vi "SubVI_Strain_test.vi"() -> (0 "error out":errorcluster caption="에러 출력", 3 "웨이브폼 차트":waveform(dbl)[](graph)=[{"t0"=timestamp(3537999110.3911605 s since 1904-01-01), "dt"=0.00062, "Y"=[0.00047262587047964, 0.00041043910651785673, 0.0005114070256648253, 0.0004353033393431034, 0.0004534332939897456, 0.000463390432462872, 0.00043454570170866036, 0.0003840550210499824, 0.00046049693560497513, 0.00043601921847729236, 0.00038526592644869665, 0.0005006792607078738, 0.00047117014412360745, 0.0004275898066649711, 0.00042875309283979117, 0.0004913538098973309, 0.00038979939141159815, 0.00047844285209712467, 0.00036011787223929454, 0.0004068360428684548, 0.0004042828942719733, 0.0004761339497591499, 0.0003612452128748545, 0.00039843694890317436, 0.0004418536716216596, 0.00036188344388491333, 0.0004565713521915321, 0.00047409353330743514, 0.00037547139637794424, 0.00033699303793574255, 0.00041919632967674477, 0.0004044857140110813, 0.0003804044274407727, 0.0004687777505846543, 0.00042779860142021844, 0.00037995705260560905, 0.0003900678215465565, 0.0004465785547122237, 0.00037223244355367514, 0.0004662123537668788, 0.00045247278961574056, 0.0003887435676117308, 0.0003601775198283073, 0.00036035646263802423, 0.0003362236202489259, 0.00044848164523168013, 0.0003231198433927978, 0.00034800359433781783, 0.0003373986229292269, 0.00041982270369339325, 0.0003728468289415956, 0.00030865658295483727, 0.0004351243697196373, 0.00039441044463494316, 0.00040742660946971977, 0.0003725068291676455, 0.00034785447900801964, 0.00036742475482860114, 0.0003175730590198825, 0.00037625876929430786, 0.00034030930135528964, 0.0002938836142782422, 0.0003432021030489953, 0.0003697689446748764, 0.0003789907243272393, 0.0002950167696174689, 0.00037915774389622395, 0.00037210121570454955, 0.0003386332733897068, 0.0004143583625068418, 0.00033167274759207834, 0.0002777215202054256, 0.00035874597965521654, 0.00037385489980525907, 0.0003248852844424059, 0.00036311815478616875, 0.0002994301359364881, 0.000380660922526737, 0.0003066943831403147, 0.00029233298481648196, 0.00039809096652279293, 0.0002827788278151317, 0.0002551908820106478, 0.0003740815669064443, 0.00027501397323419517, 0.00037588297752052364, 0.00038506311450266543, 0.00026713592984576207, 0.0003405777049319909, 0.00025879285341093864, 0.0003032650250487586, 0.0003875087934527209, 0.00035051470316939084, 0.0002406520624579295, 0.00026611018313775064, 0.0003136366687181668, 0.00036281395036811534, 0.0003465422660227054, 0.0003349531889845697, 0.00034369716151030395], "attributes"=variant("NI_ChannelName"=variant(string "Strain/ai0"), "NI_UnitDescription"=variant(string "Strain"))}, {"t0"=timestamp(3537999110.3911605 s since 1904-01-01), "dt"=0.00062, "Y"=[0.0002669331657947935, 0.00031134641952601326, 0.0002354460989940313, 0.00016687317361001626, 0.00022731822544217194, 0.00024163601353161676, 0.0002590850674601926, 0.00023137916409462781, 0.00026835251587787164, 0.00026616981951666294, 0.00017885188772679905, 0.00017816022694101572, 0.00017185781023223087, 0.00017636549091540666, 0.0002635517891786011, 0.00022700814043906276, 0.00023874379922674913, 0.00024052683246014774, 0.00024122454284711817, 0.00016479228139494308, 0.00021975697672062318, 0.00028465743977653437, 0.0001807718476799469, 0.00022712740387904418, 0.00019713950741664365, 0.0002739703191745871, 0.00017310397715106191, 0.00017920964368102032, 0.00026575236501360995, 0.00014409711692620224, 0.00016225825528964416, 0.00019742572262577832, 0.0002141517083944936, 0.00023250025135162307, 0.00022681731899424989, 0.0002503843181970984, 0.0002561748616886476, 0.00020925609458375476, 0.00011095444145538343, 0.0002301745944171381, 0.00011181890140260174, 0.00010877839372105932, 0.00010601810569876974, 0.00023378831215355343, 0.00018893474107480976, 0.00016091671725580725, 0.0001314395631869098, 0.00024415851512703387, 0.00021396089185510105, 0.0001720724607719918, 0.00016615171716228845, 0.00011148504083206682, 0.00011351801668865663, 0.00010659639372036722, 0.0002298346916171518, 0.00013468291901361026, 0.0001456949844501603, 0.00021809924188589055, 0.00021406226313258812, 0.00014225480585682522, 0.00013101029708028974, 0.00013037236063033694, 0.0001637250076583648, 7.379600007796863e-05, 0.0001839439715783761, 0.0001691389113699347, 0.0001081583708945824, 0.00011124060734140677, 9.396363549484408e-05, 0.00014283313578525048, 0.00019245871942893576, 5.996587190824817e-05, 0.00020705576732404593, 7.412983548600947e-05, 5.854711315164868e-05, 8.0228332253737e-05, 5.655608874399001e-05, 0.00018115941812987514, 0.00017679479595671208, 6.82519803505827e-05, 0.00014493778539749518, 0.00010855184682994629, 0.00017683057139345637, 8.758478021039626e-05, 0.00012452961605176617, 0.00010902878777275229, 0.00017910827946800666, 5.026116552805535e-05, 0.00012914418620521909, 0.0001243746053905065, 0.0001760554375036641, 0.00014819315323548205, 0.00015514516356190044, 6.678550799302241e-05, 0.00016331360107205736, 8.419269311144614e-05, 4.2714515443818715e-05, 0.00010017564567018714, 0.0001209763068135592, 0.00010350226250175502], "attributes"=variant("NI_ChannelName"=variant(string "Strain/ai1"), "NI_UnitDescription"=variant(string "Strain"))}, {"t0"=timestamp(3537999110.3911605 s since 1904-01-01), "dt"=0.00062, "Y"=[7.764108211699364e-05, 1.4484139330982968e-05, 0.00010107585700148278, 6.181040236646698e-06, 8.555787126842158e-05, -1.462080646377688e-05, 6.060371854331264e-05, 7.160223008400242e-05, 4.869340815177723e-05, 3.8333218719135346e-05, 2.0105052086062475e-05, 8.583143028958988e-06, -2.0879072364570083e-05, 8.161734533826009e-05, 3.134110632507873e-05, -5.908855668863389e-05, -1.764266463601186e-05, -5.6490094374337585e-05, -3.236427656186244e-05, -5.9529578768390715e-05, 1.3631768895227626e-05, 2.8605088960366313e-05, 3.01727833530734e-05, -6.644880668367357e-05, -6.587667777447305e-05, 2.3973564275569672e-05, 5.4213366584198175e-05, 5.71104749832485e-05, 1.7214118757940295e-05, 5.4776971863549126e-06, 1.532458992461321e-05, -3.504034488329816e-05, -4.5231921596921784e-05, 4.3996126504963626e-05, -6.430331989833602e-05, -6.589455681279568e-05, -3.6667435101351785e-05, -3.8342200088792025e-05, -5.96785726263405e-05, 2.0897826413855974e-05, -5.958917631689875e-05, -1.1855224004457564e-05, 1.3280092006003315e-05, -3.2638440121926624e-05, -2.9270985978232148e-05, -8.310581447828447e-05, -9.599599094708993e-05, 7.420833785214426e-06, -6.753942560329031e-05, -8.866001355790166e-05, -6.653224209489772e-05, 2.3121177662968224e-05, 3.486884085512345e-06, -3.879516047389555e-05, 5.126002383805686e-07, -9.907099088208958e-05, -3.235235640366676e-05, -6.12400255867085e-05, -6.194923352693948e-05, -0.00011208589745393728, -0.0001289916598464899, -4.500544437136647e-05, -0.00013066611559436767, -0.00010190760195845445, -7.196743317198027e-05, -3.4056936140276524e-05, -3.583303052276851e-05, -0.00013141693734695874, -2.2035352919422305e-05, -2.1081719665376785e-05, -0.00010476803380497741, -3.408673643363535e-05, -9.041943393893871e-06, -4.126855533843273e-05, -5.5751079689928154e-05, -0.00010771783700580792, -2.5605501263270295e-05, -0.00011601890695171023, -0.00014168401373086987, -0.0001582491364176448, -0.00012089341214936181, -4.6745740417333314e-05, -4.3968415765053384e-05, -4.3509500120545156e-05, -4.439157137568061e-05, -0.00010854020328056746, -0.0001660369378640863, -6.683618526089393e-05, -8.957776154292598e-05, -9.402941130561796e-05, -7.741448424702261e-05, -0.0001709764980914279, -0.0001377452473136861, -0.0001570097505522338, -0.00010712191857012992, -0.00018182071726395756, -5.1769917274699954e-05, -0.00015633642905843735, -8.77243856311545e-05, -5.209770879092542e-05], "attributes"=variant("NI_ChannelName"=variant(string "Strain/ai2"), "NI_UnitDescription"=variant(string "Strain"))}, {"t0"=timestamp(3537999110.3911605 s since 1904-01-01), "dt"=0.00062, "Y"=[-0.00020050558921099482, -0.0001495614534698621, -0.00020073199600438205, -0.00018995372727203654, -0.00012122115834862455, -0.0001212449944274623, -0.00013777504142727077, -0.00017362799098946113, -0.00012387887413806264, -0.000158088254772116, -0.00026515843648599154, -0.00020275177838660323, -0.0002680715498084084, -0.0002333394614464209, -0.00016174085122767803, -0.00014708263558971883, -0.00014394238471392306, -0.00023039039939810315, -0.0002208460429555684, -0.0001706964519530012, -0.00024042905457750266, -0.0002613278751332449, -0.00016952859828025523, -0.0001509617417915827, -0.00016466648427866543, -0.0002358953011486634, -0.00028687829613741473, -0.00014711838785804043, -0.00016017375357009668, -0.00018007493303118902, -0.00022324108585627383, -0.00026905449832580436, -0.00022592804818862385, -0.0002548819809070258, -0.00021847482002315826, -0.0002462615100112699, -0.0002850435227661144, -0.00017529038048775278, -0.00022102477789661643, -0.00019625150566059734, -0.00020357398834660039, -0.00027859197721010013, -0.0002065947046323231, -0.00019346309512085287, -0.00025896875897879083, -0.00019368354694769457, -0.0001968532759801585, -0.00028806970381102564, -0.0002592844999175345, -0.00020924600861882837, -0.0002782047626858196, -0.00022479011246728082, -0.0003115577262445993, -0.00024291336720367064, -0.00032061786294108327, -0.00021131937811807593, -0.00024083417114803055, -0.00030985409245419033, -0.0002963082101626119, -0.00033734383770658247, -0.00020860850534884222, -0.00024162653055014943, -0.00029837526166975355, -0.0002934369601682789, -0.00028180286763198747, -0.0003046240195780236, -0.0002597849191100339, -0.00028932067881207315, -0.00030155028379136924, -0.00031927761638318004, -0.0002718901450357661, -0.00032302434107461613, -0.00035175822448159307, -0.0002785026200388123, -0.00030336116917805474, -0.00034953652998153566, -0.00032803978549270237, -0.00036639257124389534, -0.0003688405214832027, -0.0002995428143629439, -0.0002563177187015114, -0.0003773278473498443, -0.00024785812537499906, -0.000248054723182829, -0.00031152794248694377, -0.00033438347624261083, -0.00025311857946685426, -0.0002833040560781859, -0.00038667267312756835, -0.00035811352660563997, -0.00034979860705829563, -0.0003755053179466738, -0.00026142915007245255, -0.00038550532394399296, -0.0003241560965871479, -0.0003956063776242869, -0.0003704546135005458, -0.00033861255868094153, -0.00040193729953294516, -0.00028397124949602193], "attributes"=variant("NI_ChannelName"=variant(string "Strain/ai3"), "NI_UnitDescription"=variant(string "Strain"))}])   [LabVIEW 2016]
uses:
  <vilib>/Utility/error.llb/DialogType.ctl
  <vilib>/DAQmx/read.llb/DAQmx Read (Analog 1D Wfm NChan NSamp).vi
  <vilib>/DAQmx/create/channels.llb/DAQmx Create Channel (AI-Strain-Strain Gage).vi
  <vilib>/DAQmx/configure/timing.llb/DAQmx Timing (Sample Clock).vi
  <vilib>/DAQmx/configure/task.llb/DAQmx Configure Logging (TDMS).vi
  <vilib>/DAQmx/configure/trigger.llb/DAQmx Start Trigger (Digital Edge).vi
  <vilib>/DAQmx/configure/trigger.llb/DAQmx Start Trigger (Analog Edge).vi
  <vilib>/DAQmx/calibration/calibrationInfo.llb/DAQmx Perform Shunt Calibration Ex (Strain).vi
  <vilib>/DAQmx/miscellaneous.llb/DAQmx Fill In Error Info.vi
  <resource>/objmgr/daqmx.rc
panel:
  in  "스트레인 게이지 정보":T1={"게이지 인자"=2.0, "공칭 게이지 저항"=120.0, "포와송 비"=0.3} {"공칭 게이지 저항" format="%0.2f"; "포와송 비" format="%0.2f"; "게이지 인자" format="%0.2f"}
  in  "브리지 정보":T2={"변형률 설정"=10271, "도선 저항"=0.0, "초기 브리지 전압"=0.0, "전압 구동 소스"=10200, "전압 구동 값"=2.5} {"초기 브리지 전압" format="%0.2f"; "전압 구동 소스" items=["내부"=10200, "외부"=10167, "없음"=10230]; "전압 구동 값" format="%0.2f"; "도선 저항" format="%0.2f"; "변형률 설정" items=["완전 브리지 I"=10183, "완전 브리지 II"=10184, "완전 브리지 III"=10185, "반 브리지 I"=10188, "반 브리지 II"=10189, "쿼터 브리지 I"=10271, "쿼터 브리지 II"=10272]}
  in  "TDMS 파일 경로":path
  in  "로깅 모드":i32(ring)=10231 items=["Off"=10231, "로그 및 읽기"=15842]
  in  "트리거 타입":T3(tab)
  in  "에지":i32(ring)=10280 items=["상승"=10280, "하강"=10171]
  in  "디지털 트리거 소스":tag
  in  "레벨(V)":dbl format="%0.2f"
  in  "히스테리시스(V)":dbl
  in  "기울기":i32(ring)=10280 items=["상승"=10280, "하강"=10171]
  in  "아날로그 트리거 소스":string="APFI0"
  in  "일시 정지 시점":i32(ring)=10192 items=["높음"=10192, "낮음"=10214]
  in  "일시 정지 트리거 소스":tag
  in  "샘플 클럭 소스":tag="OnboardClock"
  in  "분기 저항":dbl=100000.0 format="%#.3p"
  in  "분기 원소 위치":i32(ring)=12465 items=["R1"=12465, "R2"=12466, "R3"=12467, "R4"=14813, "없음"=10230]
  in  "분기 교정 수행?":bool caption="분기 교정 활성화"
  in  "오프셋 널 수행?":bool caption="오프셋 널 활성화"
  in  "최대값":dbl=0.001
  in  "최소값":dbl=-0.001
  in  "물리적인 채널":tag="Strain/ai0:3"
  in  "샘플 속도":dbl=50000.0
  out "실제 샘플 속도":dbl=1612.9032258064517 format="%0.2f"
  in  "루프 당 샘플":i32=1000
  in  "정지":bool
  # "시작 트리거를 설정하고 사용하려면 위의 탭이 있어야 합니다.   일부 하드웨어는 트리거를 지원하지 않습니다. 더 자세한 정보는 디바이스 문서를 참조하십시오."
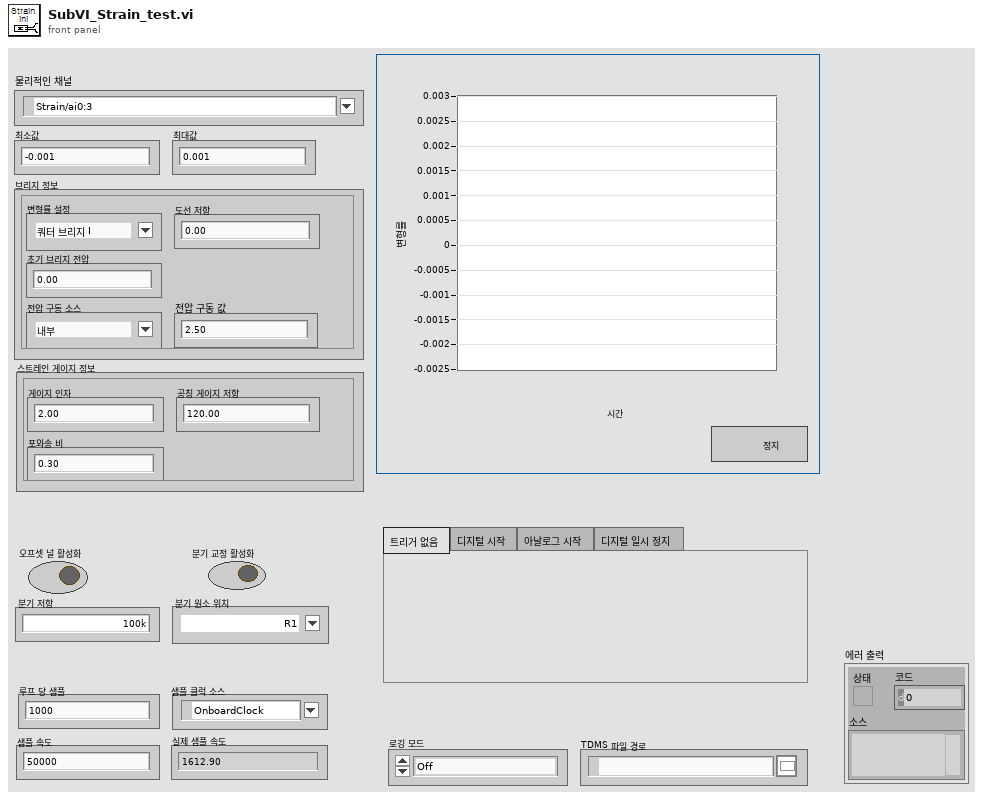
[diagram p1: front panel]
types:
  T1 = cluster{"게이지 인자":dbl, "공칭 게이지 저항":dbl, "포와송 비":dbl}
  T2 = cluster{"변형률 설정":i32, "도선 저항":dbl, "초기 브리지 전압":dbl, "전압 구동 소스":i32, "전압 구동 값":dbl}
  T3 = enum32{"No Trigger", "Digital Start", "Analog Start", "Digital Pause"}
  T4 = typedef "DialogType.ctl" = u16
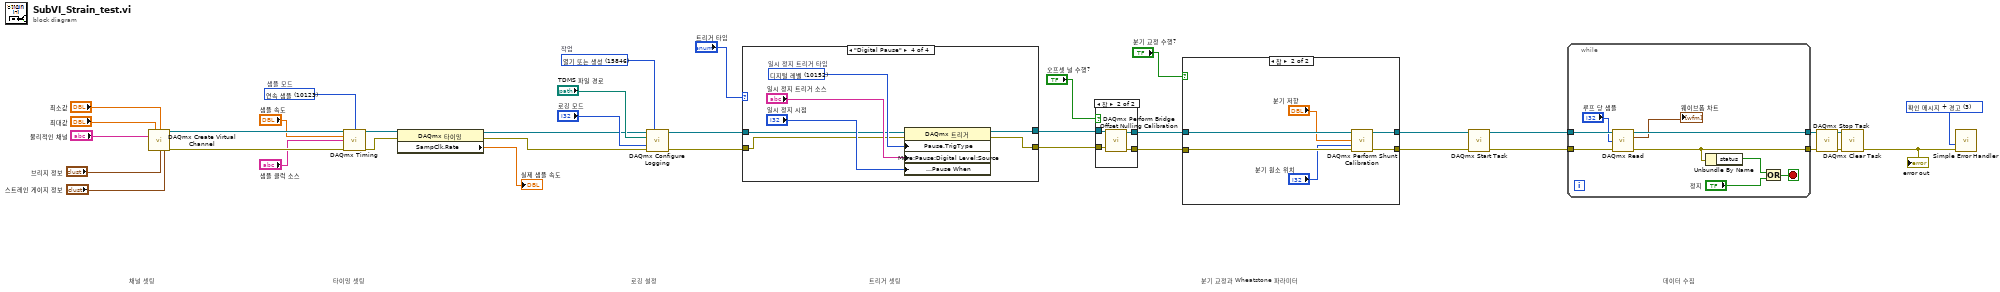
[diagram p0: block diagram]
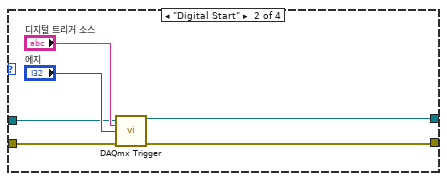
[diagram p3: hidden frame]
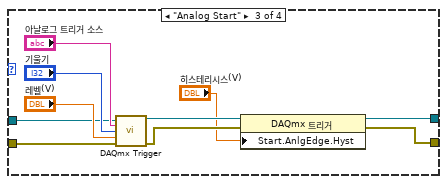
[diagram p4: hidden frame]
diagram:
  w1 = T4 3 items=["대화 상자 없음", "확인 메시지", "메시지 지속 또는 정지", "확인 메시지 + 경고", "지속/정지 + 경고"] ("대화 상자 타입 (확인 메시지:1)")
  w12 = 15846 items=["열기"=10437, "열기 또는 생성"=15846, "생성 또는 대체"=15847, "생성"=15848]  # 작업
  w35 = 10123 items=["유한 샘플"=10178, "연속 샘플"=10123, "하드웨어 타이밍에 의한 단일 포인트"=12522]  # 샘플 모드
  # "로깅 설정"
  # "트리거 셋팅"
  # "데이터 수집"
  # "분기 교정과 Wheatstone 파라미터"
  # "타이밍 셋팅"
  # "채널 셋팅"
  n1 = call-poly <vilib>:"DAQmx Create Virtual Channel.vi"("maximum value"="최대값", "minimum value"="최소값", "physical channels"="물리적인 채널", "bridge information"="브리지 정보", "strain gage information"="스트레인 게이지 정보") -> ("task out"=w33:refnum<k21>, "error out"=w34:errorcluster)  [unwired: 9 in]
  n2 = call-poly <vilib>:"DAQmx Timing.vi"("task/channels in"=w33, "sample mode"=w35, "rate"="샘플 속도", "source"="샘플 클럭 소스", "error in"=w34) -> ("task out"=w37:refnum<k21>, "error out"=w36:errorcluster)  [unwired: 9 in]
  n3 = property class="DAQmx 타이밍"(reference=w37, error in=w36) -> (reference out=w11:refnum<k21>, error out=w10:errorcluster, "SampClk.Rate"=→"실제 샘플 속도":dbl)
  n4 = call-poly <vilib>:"DAQmx Configure Logging.vi"("task/channels in"=w11, "operation"=w12, "file path"="TDMS 파일 경로", "logging mode"="로깅 모드", "error in"=w10) -> ("task out"=w9:refnum<k21>, "error out"=w8:errorcluster)  [unwired: 9 in]
  n5 = case shown="\"Digital Pause\"" "트리거 타입" {
    tunnel: [w39 w45 w54 w62] -> w18
    tunnel: [w38 w44 w53 w61] -> w17
    tunnel: w9 -> [w39 w41 w47 w57]
    tunnel: w8 -> [w38 w40 w46 w56]
    frame "No Trigger", Default {
    }
    frame "Digital Start" {
      n6 = call-poly <vilib>:"DAQmx Trigger.vi"("task/channels in"=w41, "source"="디지털 트리거 소스", "edge"="에지", "error in"=w40) -> ("task out"=w45:refnum<k21>, "error out"=w44:errorcluster)  [unwired: 10 in]
    }
    frame "Analog Start" {
      n7 = call-poly <vilib>:"DAQmx Trigger.vi"("task/channels in"=w47, "source"="아날로그 트리거 소스", "slope"="기울기", "level"="레벨(V)", "error in"=w46) -> ("task out"=w52:refnum<k21>, "error out"=w51:errorcluster)  [unwired: 9 in]
      n8 = property class="DAQmx 트리거"(reference=w52, error in=w51, "Start.AnlgEdge.Hyst"="히스테리시스(V)") -> (reference out=w54:refnum<k21>, error out=w53:errorcluster)
    }
    frame "Digital Pause" {
      w60 = 10152 items=["아날로그 레벨"=10101, "아날로그 윈도우"=10103, "디지털 레벨"=10152, "디지털 패턴"=10398, "없음"=10230]  # 일시 정지 트리거 타입
      n9 = property class="DAQmx 트리거"(reference=w57, error in=w56, "Pause.TrigType"=w60, "More:Pause:Digital Level:Source"="일시 정지 트리거 소스", "More:Pause:Digital Level:Pause When"="일시 정지 시점") -> (reference out=w62:refnum<k21>, error out=w61:errorcluster)
    }
  }
  n10 = case shown="참" "오프셋 널 수행?" {
    tunnel: [w64 w68] -> w23
    tunnel: [w63 w67] -> w22
    tunnel: w18 -> [w64 w66]
    tunnel: w17 -> [w63 w65]
    frame False {
    }
    frame True {
      n11 = call <vilib>:"DAQmx Perform Bridge Offset Nulling Calibration.vi"("task/channels in"=w66, "error in"=w65) -> ("task out"=w68:refnum<k21>, "error out"=w67:errorcluster)  [unwired: 12 in]
    }
  }
  n12 = case shown="참" "분기 교정 수행?" {
    tunnel: w23 -> [w70 w76]
    tunnel: w22 -> [w69 w75]
    tunnel: [w69 w74] -> w15
    tunnel: [w70 w73] -> w16
    frame False {
    }
    frame True {
      n13 = call-poly <vilib>:"DAQmx Perform Shunt Calibration.vi"("task/channels in"=w76, "shunt resistance"="분기 저항", "shunt element location"="분기 원소 위치", "error in"=w75) -> ("task out"=w73:refnum<k21>, "error out"=w74:errorcluster)  [unwired: 10 in]
    }
  }
  n14 = call <vilib>:"DAQmx Start Task.vi"("task/channels in"=w16, "error in"=w15) -> ("task out"=w32:refnum<k21>, "error out"=w31:errorcluster)  [unwired: 12 in]
  n15 = while {
    tunnel: w32 -> [w85]
    tunnel: w31 -> [w84]
    tunnel: [w81] -> w3
    tunnel: [w82] -> w4
    stop <- w83 stop-if-true
    n16 = call-poly <vilib>:"DAQmx Read.vi"("task/channels in"=w85, "number of samples per channel"="루프 당 샘플", "error in"=w84) -> ("task out"=w82:refnum<k21>, "data"=→"웨이브폼 차트":waveform(dbl)[], "error out"=w81:errorcluster)  [unwired: 10 in]
    n17 = Unbundle By Name(w81) -> ("status"=w80:bool)
    n18 = Or(x=w80, y="정지") -> (x .or. y?=w83:bool)
  }
  n19 = call <vilib>:"DAQmx Stop Task.vi"("task/channels in"=w4, "error in"=w3) -> ("task out"=w5:refnum<k21>, "error out"=w2:errorcluster)  [unwired: 12 in]
  n20 = call <vilib>:"DAQmx Clear Task.vi"("task in"=w5, "error in"=w2) -> ("error out"=w30:errorcluster)  [unwired: 13 in]
  "error out" <- w30
  n21 = call <vilib>:"Simple Error Handler.vi"("type of dialog (OK msg:1)"=w1, "error in (no error)"=w30) -> ()  [unwired: 3 in, 5 out]
